vi "acquireManualControlActiveSignal.vi"(8 "error in (no error)":errorcluster, 11 "cRIOScanModeTarget in":refnum<class "cRIOScanModeTarget.lvclass">) -> (0 "error out":errorcluster, 2 "manualControlActiveIsT":bool, 3 "cRIOScanModeTarget out":refnum<class "cRIOScanModeTarget.lvclass">)   [LabVIEW 2012, in "cRIOScanModeTarget.lvclass"]
doc: "Acquires the value of the manual control active signal for the systems. (There is presently a single signal that applies to all elements on the device.)"
uses:
  cRIOScanModeTarget.lvclass
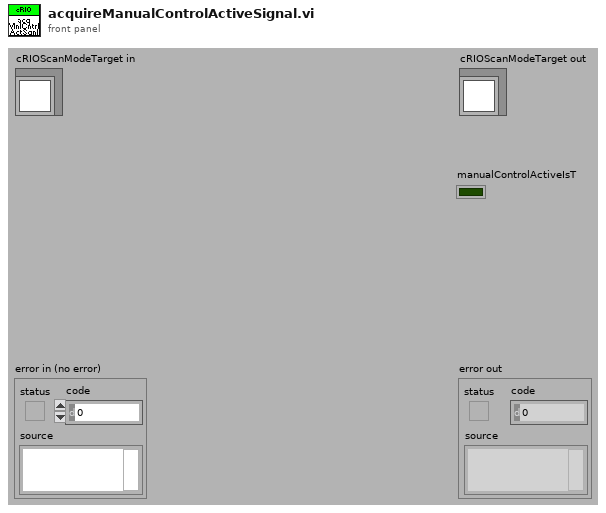
[diagram p1: front panel]
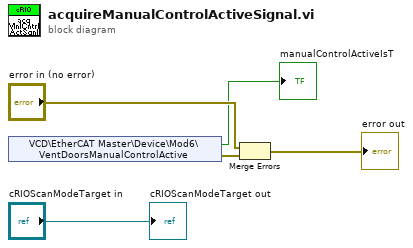
[diagram p0: block diagram]
diagram:
  n1 = shared-variable "VCD\\EtherCAT Master\\Device\\Mod6\\VentDoorsManualControlActive"() -> (→"manualControlActiveIsT":bool, error out=w1:errorcluster)  [unwired: 1 in]
  n2 = Merge Errors("error in (no error)", w1) -> (→"error out":errorcluster)
  "cRIOScanModeTarget out" <- "cRIOScanModeTarget in"
